vi "startShooting.vi"(8 "error in (no error)":errorcluster, 11 "CameraController in":refnum<class "CameraController.lvclass">) -> (0 "error out":errorcluster, 1 "Warning Message":string, 2 "Final Acquisition Timings":T1, 3 "CameraController out":refnum<class "CameraController.lvclass">)   [LabVIEW 2009, in "Hardware.lvlib" / "Channels.lvlib" / "CameraController.lvclass"]
uses:
  CameraController.lvclass
  CameraAcquisitor.lvclass
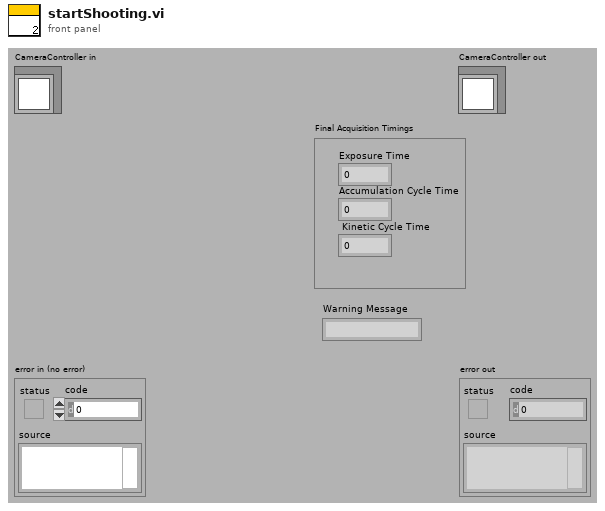
[diagram p1: front panel]
types:
  T1 = cluster{"Exposure Time":dbl, "Accumulation Cycle Time":dbl, " Kinetic Cycle Time":dbl}
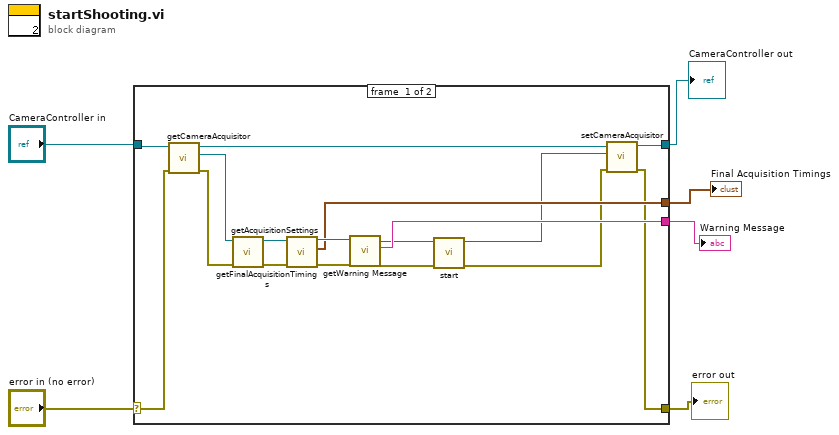
[diagram p0: block diagram]
diagram:
  n1 = case shown="No Error" "error in (no error)" {
    selector: "error in (no error)" -> [w22 w25]
    tunnel: [w7 w25] -> w5
    tunnel: [w8 w24] -> w3
    tunnel: "CameraController in" -> [w23 w24]
    tunnel: [w15 _] -> w2
    tunnel: [w14 _] -> w1
    frame #0 {
      n2 = call-dynamic "getCameraAcquisitor.vi"("error in (no error)"=w22, "CameraController.lvclass in"=w23) -> ("error out"=w16:errorcluster, "CameraAcquisitor.lvclass"=w17:refnum<class "CameraAcquisitor.lvclass">, "CameraController.lvclass out"=w11:refnum<class "CameraController.lvclass">)  [unwired: 7 in]
      n3 = call-dynamic "getAcquisitionSettings.vi"("error in (no error)"=w16, "CameraAcquisitor in"=w17) -> ("error out"=w20:errorcluster, "CameraAcquisitor out"=w21:refnum<class "CameraAcquisitor.lvclass">)  [unwired: 8 in]
      n4 = call-dynamic "getFinalAcquisitionTimings.vi"("error in (no error)"=w20, "CameraAcquisitor.lvclass in"=w21) -> ("error out"=w18:errorcluster, "Final Acquisition Timings"=w15:T1, "CameraAcquisitor.lvclass out"=w19:refnum<class "CameraAcquisitor.lvclass">)  [unwired: 7 in]
      n5 = call-dynamic "getWarning Message.vi"("error in (no error)"=w18, "CameraAcquisitor.lvclass in"=w19) -> ("error out"=w13:errorcluster, "Warning Message"=w14:string, "CameraAcquisitor.lvclass out"=w12:refnum<class "CameraAcquisitor.lvclass">)  [unwired: 7 in]
      n6 = call-dynamic "start.vi"("error in (no error)"=w13, "CameraAcquisitor in"=w12) -> ("error out"=w9:errorcluster, "CameraAcquisitor out"=w10:refnum<class "CameraAcquisitor.lvclass">)  [unwired: 8 in]
      n7 = call-dynamic "setCameraAcquisitor.vi"("error in (no error)"=w9, "Hardware:Channels.lvlib:CameraAcquisitor.lvclass"=w10, "CameraController.lvclass in"=w11) -> ("error out"=w7:errorcluster, "CameraController.lvclass out"=w8:refnum<class "CameraController.lvclass">)  [unwired: 7 in]
    }
    frame #1 {
    }
  }
  "error out" <- w5
  "CameraController out" <- w3
  "Final Acquisition Timings" <- w2
  "Warning Message" <- w1
